vi "CreateParameterIndexArray.vi"(10 "length":i32, 11 "list":string) -> (3 "Array":i32[](array[numeric]))   [LabVIEW 2014, in "Raspberry Pi Compatible Compiler for LabVIEW.lvlib" / "Python Functions.lvlib"]
uses:
  Python Functions.lvlib
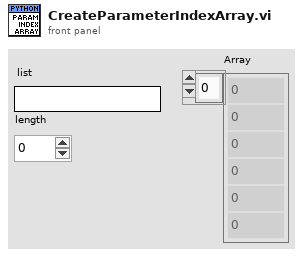
[diagram p1: front panel]
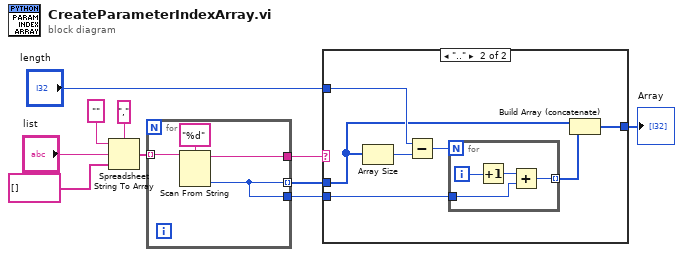
[diagram p0: block diagram]
diagram:
  n1 = Spreadsheet String To Array(delimiter (Tab)=",", format string="", spreadsheet string="list", array type (2D Dbl)=string[] []) -> (array=w7:string[])
  n2 = for {
    tunnel: w7 -> [w14] mode=indexing
    tunnel: [w12] -> w6
    tunnel: [w11] -> w5
    tunnel: [w11] -> w4 mode=indexing
    n3 = Scan From String(format string="%d", input string=w14) -> (remaining string=w12:string, output 1=w11:i32)  [unwired: 3 in, 2 out]
  }
  n4 = case shown="\"..\"" w6 {
    tunnel: w5 -> [_ w19]
    tunnel: w4 -> [w15 w18]
    tunnel: "length" -> [_ w21]
    tunnel: [w15 w16] -> w2
    frame Default {
    }
    frame ".." {
      n5 = Array Size(array=w18) -> (size(s)=w22:i32)
      n6 = Subtract(x=w21, y=w22) -> (x-y=w20:i32)
      n7 = for {
        N: w20 -> [_]
        tunnel: w19 -> [w24]
        tunnel: [w23] -> w17 mode=indexing
        i -> [w26]
        n8 = Increment(x=w26) -> (x+1=w25:i32)
        n9 = Add(x=w25, y=w24) -> (x+y=w23:i32)
      }
      n10 = Build Array (concatenate)(w18, w17) -> (w16:i32[])
    }
  }
  "Array" <- w2
